vi "SRS865A--set--freq--V1.vi"(8 "error in (no error)":errorcluster, 9 "freq in":dbl, 11 "VISA resource name":refnum<visa-resource-name>) -> (0 "error out":errorcluster, 1 "freq out":dbl, 2 "zi out (V)":cdb, 3 "VISA resource name out":refnum<visa-resource-name>)   [LabVIEW 2017]
uses:
  <instrlib>/Stanford Research SR865/Stanford Research SR865.lvlib
panel:
  out "concatenated string":string
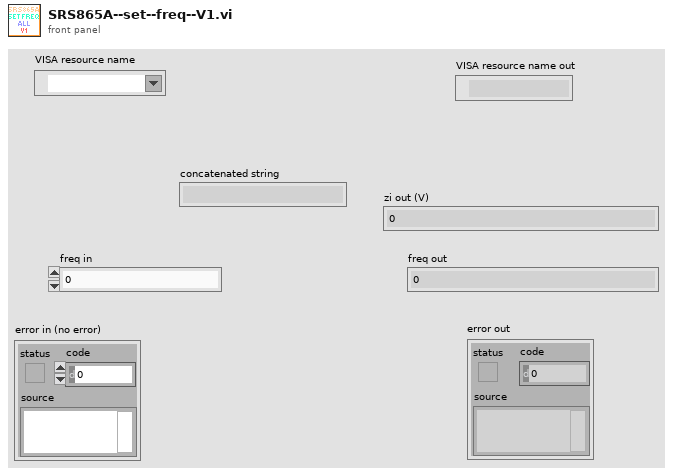
[diagram p1: front panel]
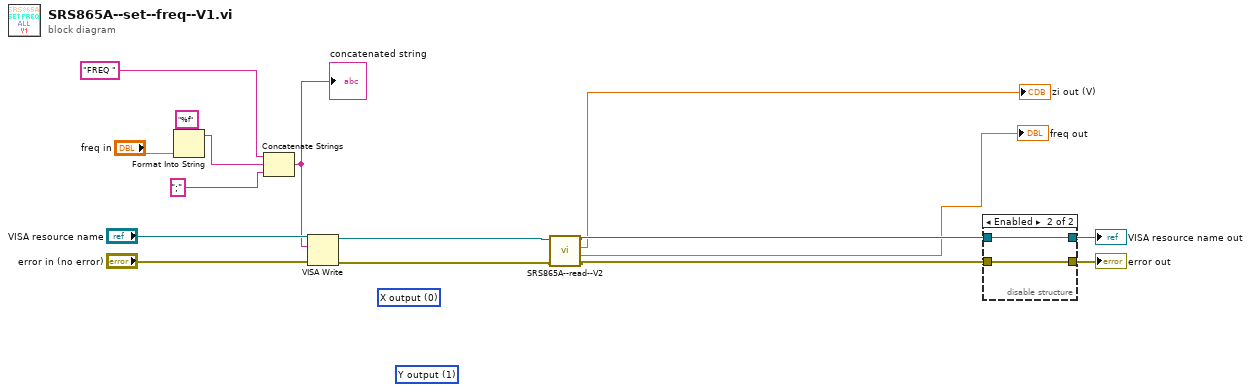
[diagram p0: block diagram]
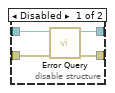
[diagram p2: hidden frame]
diagram:
  (unwired) 1 items=["X output", "Y output", "R output", "Theta output", "Aux In 1", "Aux In 2", "Aux In 3", "Aux In 4", "Aux Out 1", "Aux Out 2", "Xnoise", "Ynoise", "Reference Phase", "Sine Out Amplitude", "DC Level", "Int. Ref. Frequency", "Ext. Ref. Frequency"] ("Single Lock-in Parameter 2 (0: X output)")
  (unwired) 0 items=["X output", "Y output", "R output", "Theta output", "Aux In 1", "Aux In 2", "Aux In 3", "Aux In 4", "Aux Out 1", "Aux Out 2", "Xnoise", "Ynoise", "Reference Phase", "Sine Out Amplitude", "DC Level", "Int. Ref. Frequency", "Ext. Ref. Frequency"] ("Single Lock-in Parameter 1 (0: X output)")
  n1 = Format Into String(format string="%f", "freq in") -> (resulting string=w10:string)  [unwired: 2 in, 1 out]
  n2 = Concatenate Strings("FREQ ", w10, ";" ("format string")) -> (w8:string)
  "concatenated string" <- w8
  n3 = VISA Write(VISA resource name="VISA resource name", write buffer=w8, error in (no error)="error in (no error)") -> (VISA resource name out=w7:refnum<visa-resource-name>, error out=w6:errorcluster)  [unwired: 1 out]
  n4 = call "SRS865A--read--V2.vi"("error in (no error)"=w6, "VISA resource name"=w7) -> ("error out"=w5:errorcluster, "freq out"=→"freq out":dbl, "zi out (V)"=→"zi out (V)":cdb, "VISA resource name out"=w4:refnum<visa-resource-name>)  [unwired: 6 in]
  n5 = disable-structure shown="Enabled" {
    disable-tunnel: [w20 w22] -> w16
    disable-tunnel: [w19 w21] -> w15
    disable-tunnel: w4 -> [w18 w22]
    disable-tunnel: w5 -> [w17 w21]
    frame Disabled {
      n6 = call <instrlib>:"Error Query.vi"("error in (no error)"=w17, "VISA resource name"=w18) -> ("error out"=w19:errorcluster, "VISA resource name out"=w20:refnum<visa-resource-name>)  [unwired: 7 in, 1 out]
    }
    frame Enabled {
    }
  }
  "VISA resource name out" <- w16
  "error out" <- w15
